vi "Populate Database Table.vi"() -> ()   [LabVIEW 2019]
uses:
  Controls/Table Data Types/Inventory Data Type.ctl
  Controls/Table Data Types/User Data Type.ctl
  Controls/Table Data Types/Inventory Archive Data Type.ctl
  Controls/Table Data Types/User Archive Data Type.ctl
  Controls/Table Data Types/Checked In Archive Data Type.ctl
  <vilib>/addons/database/Connection.llb/DB Tools Open Connec (String).vi
  <vilib>/Utility/file.llb/Read Delimited Spreadsheet (string).vi
  <vilib>/addons/database/NI_Database_API.lvlib
panel:
  in  "Checked In TXT File":path
  in  "User Archive TXT File":path
  in  "Inventory Archive TXT File":path
  in  "User TXT File":path
  in  "Inventory TXT File":path
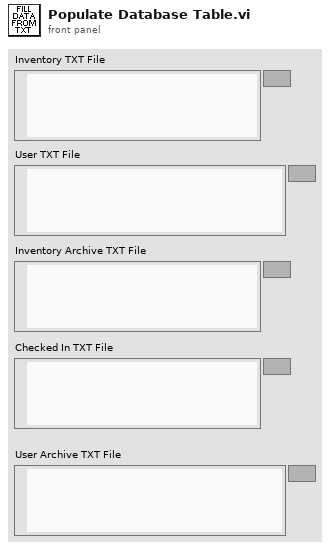
[diagram p1: front panel]
types:
  T1 = typedef "NI_Database_API.lvlib/Conn ObjectReference.ctl" = refnum<k1>
  T2 = typedef "Inventory Data Type.ctl" = cluster{"Identifier":string, "BYU ICN #":string, "Item Description":string, "Comments":string, "Checked Out Date":string, "Due Date":string, "Check Out Location":string, "Reminder Count":i32, "Most Recent Reminder Date":string, "BYU ID #":string, "Building/Room":string, "Location in Room":string, "Manual":string, "Manufacturer":string, "Model #":string, "Serial #":string, "Date Acquired":string}
  T3 = typedef "User Data Type.ctl" = cluster{"BYU ID #":string, "First Name":string, "Last Name":string, "Phone Number":string, "Email":string, "Department":string, "Graduation Status":string, "Anticipated Graduation Year":string, "Credit Score":dbl, "Date Added":string, "Graduation Clearance Date":string, "Picture File Name":string}
  T4 = typedef "Inventory Archive Data Type.ctl" = cluster{"Date Disposed":string, "Disposal Method":string, "Auction #":string, "Date Inventory Office Emailed":string, "Disposal Notes":string, "Identifier":string, "BYU ICN #":string, "Item Description":string, "Comments":string, "Building/Room":string, "Location in Room":string, "Manual":string, "Manufacturer":string, "Model #":string, "Serial #":string, "Date Acquired":string}
  T5 = typedef "User Archive Data Type.ctl" = cluster{"BYU ID #":string, "First Name":string, "Last Name":string, "Phone Number":string, "Email":string, "Department":string, "Graduation Status":string, "Anticipated Graduation Year":string, "Credit Score":dbl, "Date Added":string, "Graduation Clearance Date":string, "Picture File Name":string, "Date Archived":string}
  T6 = typedef "Checked In Archive Data Type.ctl" = cluster{"Identifier":string, "BYU ICN #":string, "Item Description":string, "Comments":string, "Checked Out Date":string, "Due Date":string, "Check Out Location":string, "Reminder Count":i32, "Most Recent Reminder Date":string, "BYU ID #":string, "Building/Room":string, "Location in Room":string, "Manual":string, "Manufacturer":string, "Model #":string, "Serial #":string, "Date Acquired":string, "Date Returned":string}
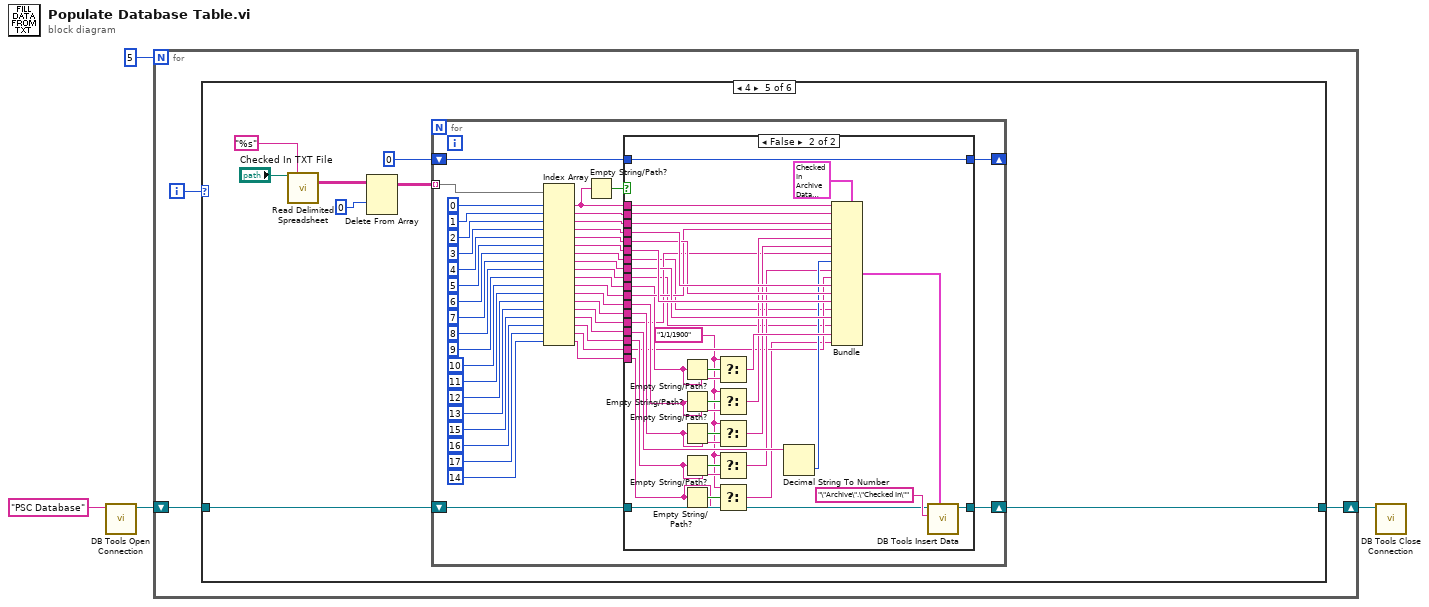
[diagram p0: block diagram]
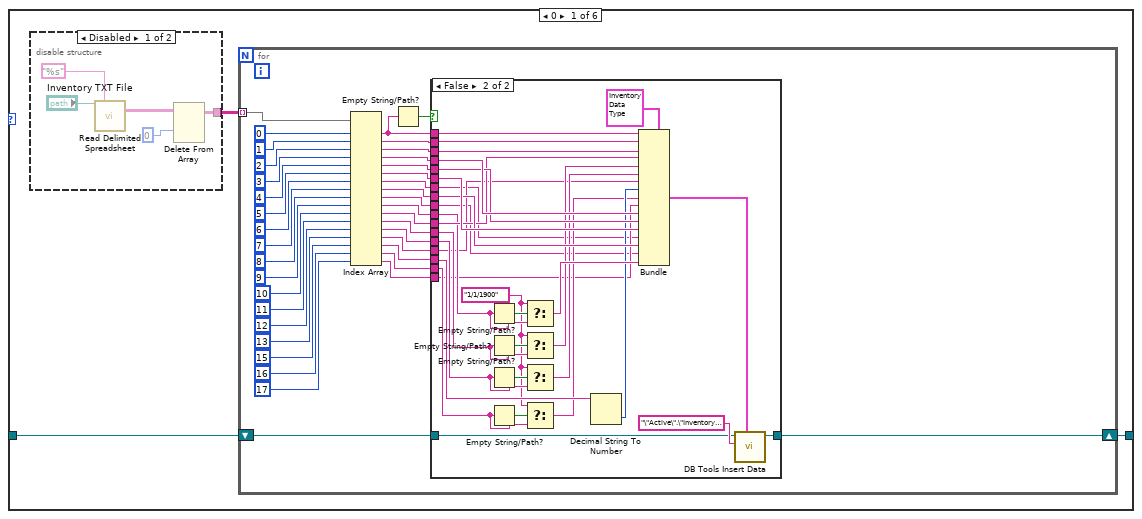
[diagram p2: hidden frame]
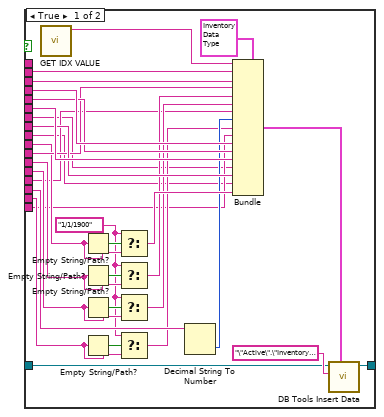
[diagram p4: hidden frame]
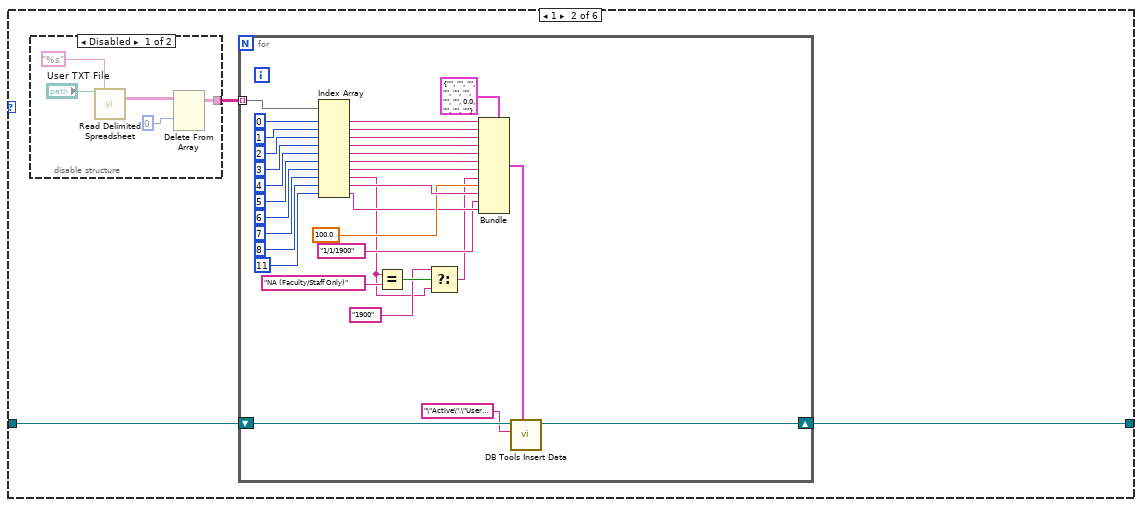
[diagram p5: hidden frame]
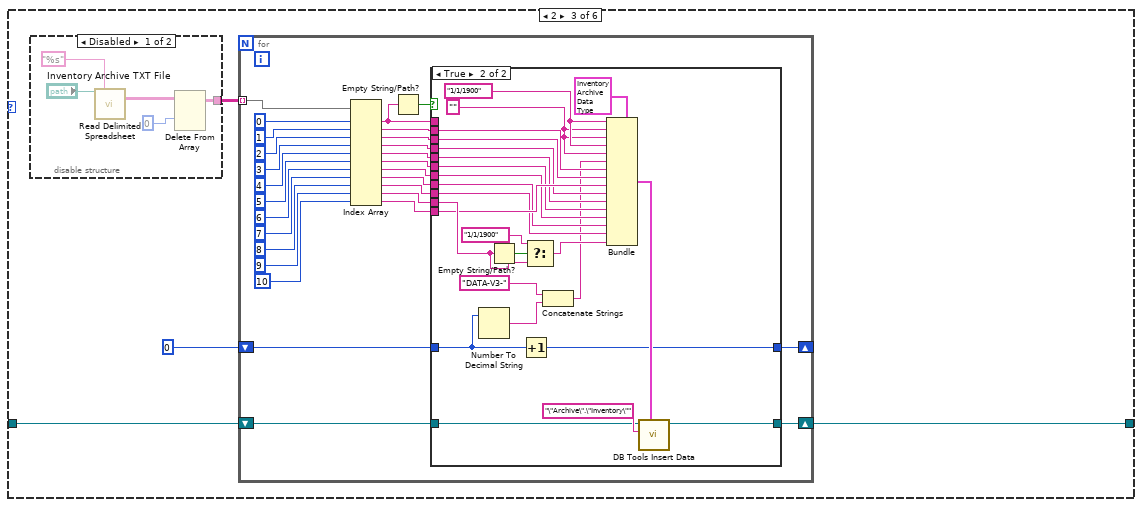
[diagram p7: hidden frame]
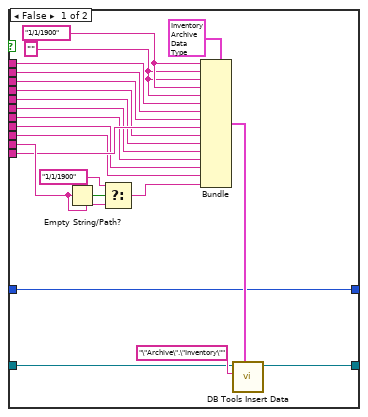
[diagram p9: hidden frame]
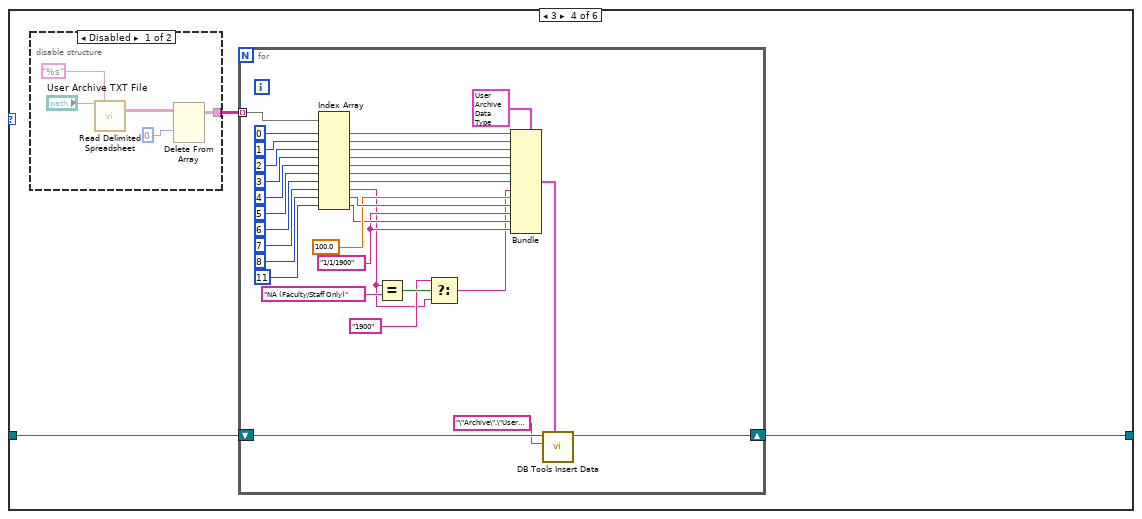
[diagram p10: hidden frame]
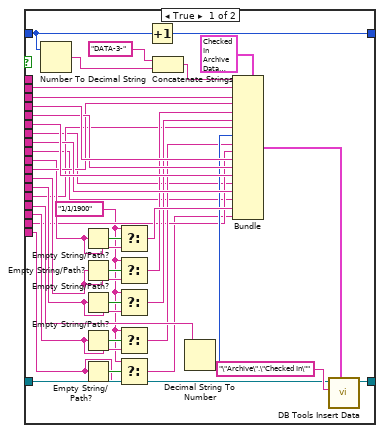
[diagram p12: hidden frame]
diagram:
  n1 = call-poly <vilib>:"DB Tools Open Connection.vi"("connection information"="PSC Database") -> ("connection reference"=w3:T1)  [unwired: 7 in, 1 out]
  n2 = for {
    N: 5 -> [_]
    shift-right: [w5] -> w1
    shift-left: w3 -> [w7]
    i -> [w6]
    n3 = case shown="4" w6 {
      tunnel: w7 -> [w10 w120 w161 w244 w287 w407]
      tunnel: [w9 w119 w160 w243 w286 w407] -> w5
      frame 0 {
        n4 = disable-structure shown="Disabled" {
          disable-tunnel: [w11 _] -> w8
          frame Disabled {
            n5 = call-poly <vilib>:"Read Delimited Spreadsheet.vi"("file path (dialog if empty)"="Inventory TXT File", "format (%s)"="%s") -> ("all rows"=w12:string[][])  [unwired: 8 in, 5 out]
            n6 = Delete From Array(array=w12, index (row)=0) -> (array with subset deleted=w11:string[][])  [unwired: 2 in, 1 out]
          }
          frame Enabled {
          }
        }
        n7 = for {
          tunnel: w8 -> [w53] mode=indexing
          shift-right: [w16] -> w9
          shift-left: w10 -> [w34]
          n8 = Index Array(array=w53, index #1=0 ("index"), index #2=1 ("index"), index #3=2 ("index"), index #4=3 ("index"), index #5=4 ("index"), index #6=5 ("index"), index #7=6 ("index"), index #8=7 ("index"), index #9=8 ("index"), index #10=9 ("index"), index #11=10 ("index"), index #12=11 ("index"), index #13=12 ("index"), index #14=13 ("index"), index #15=15 ("index"), index #16=16 ("index"), index #17=17 ("index")) -> (element #1=w27:string, element #2=w33:string, element #3=w32:string, element #4=w31:string, element #5=w30:string, element #6=w29:string, element #7=w28:string, element #8=w26:string, element #9=w25:string, element #10=w24:string, element #11=w23:string, element #12=w22:string, element #13=w21:string, element #14=w20:string, element #15=w19:string, element #16=w18:string, element #17=w17:string)
          n9 = Empty String/Path?(string/path=w27) -> (empty?=w35:bool)
          n10 = case shown="False" w35 {
            tunnel: w34 -> [w55 w88]
            tunnel: w33 -> [w83 w115]
            tunnel: w32 -> [w82 w114]
            tunnel: w31 -> [w81 w113]
            tunnel: w30 -> [w80 w112]
            tunnel: w29 -> [w79 w111]
            tunnel: w28 -> [w57 w90]
            tunnel: w27 -> [_ w87]
            tunnel: w26 -> [w78 w110]
            tunnel: w25 -> [w58 w91]
            tunnel: w24 -> [w74 w107]
            tunnel: w23 -> [w76 w109]
            tunnel: w22 -> [w72 w105]
            tunnel: w21 -> [w70 w103]
            tunnel: w20 -> [w66 w99]
            tunnel: w19 -> [w65 w98]
            tunnel: w18 -> [w62 w95]
            tunnel: w17 -> [w59 w92]
            tunnel: [w54 w86] -> w16
            frame True {
              w61 = "1/1/1900"
              n11 = call "GET IDX VALUE.vi"() -> ("Identifier Out"=w77:string)  [unwired: 11 in]
              n12 = Empty String/Path?(string/path=w74) -> (empty?=w75:bool)
              n13 = Empty String/Path?(string/path=w72) -> (empty?=w73:bool)
              n14 = Empty String/Path?(string/path=w70) -> (empty?=w71:bool)
              n15 = Empty String/Path?(string/path=w62) -> (empty?=w63:bool)
              n16 = Select(t=w61, s=w75, f=w74) -> (s? t:f=w69:string)
              n17 = Select(t=w61, s=w73, f=w72) -> (s? t:f=w68:string)
              n18 = Select(t=w61, s=w71, f=w70) -> (s? t:f=w67:string)
              n19 = Select(t=w61, s=w63, f=w62) -> (s? t:f=w60:string)
              n20 = Decimal String To Number(string=w65) -> (number=w64:i32)  [unwired: 2 in, 1 out]
              n21 = Bundle(cluster=T2 {"Identifier"="", "BYU ICN #"="", "Item Description"="", "Comments"="", "Checked Out Date"="", "Due Date"="", "Check Out Location"="", "Reminder Count"=0, "Most Recent Reminder Date"="", "BYU ID #"="", "Building/Room"="", "Location in Room"="", "Manual"="", "Manufacturer"="", "Model #"="", "Serial #"="", "Date Acquired"=""} ("INVENTORY DATA TYPE"), "Identifier"=w77, "BYU ICN #"=w83, "Item Description"=w82, "Comments"=w76, "Checked Out Date"=w68, "Due Date"=w67, "Check Out Location"=w66, "Reminder Count"=w64, "Most Recent Reminder Date"=w60, "BYU ID #"=w59, "Building/Room"=w81, "Location in Room"=w80, "Manual"=w79, "Manufacturer"=w57, "Model #"=w78, "Serial #"=w58, "Date Acquired"=w69) -> (w56:T2)
              n22 = call <vilib>:"DB Tools Insert Data.vi"("data"=w56, "table"="\"Active\".\"Inventory\"", "connection reference"=w55) -> ("connection reference out"=w54:T1)  [unwired: 7 in, 1 out]
            }
            frame False {
              w94 = "1/1/1900"
              n23 = Empty String/Path?(string/path=w107) -> (empty?=w108:bool)
              n24 = Empty String/Path?(string/path=w105) -> (empty?=w106:bool)
              n25 = Empty String/Path?(string/path=w103) -> (empty?=w104:bool)
              n26 = Empty String/Path?(string/path=w95) -> (empty?=w96:bool)
              n27 = Select(t=w94, s=w108, f=w107) -> (s? t:f=w102:string)
              n28 = Select(t=w94, s=w106, f=w105) -> (s? t:f=w101:string)
              n29 = Select(t=w94, s=w104, f=w103) -> (s? t:f=w100:string)
              n30 = Select(t=w94, s=w96, f=w95) -> (s? t:f=w93:string)
              n31 = Decimal String To Number(string=w98) -> (number=w97:i32)  [unwired: 2 in, 1 out]
              n32 = Bundle(cluster=T2 {"Identifier"="", "BYU ICN #"="", "Item Description"="", "Comments"="", "Checked Out Date"="", "Due Date"="", "Check Out Location"="", "Reminder Count"=0, "Most Recent Reminder Date"="", "BYU ID #"="", "Building/Room"="", "Location in Room"="", "Manual"="", "Manufacturer"="", "Model #"="", "Serial #"="", "Date Acquired"=""} ("INVENTORY DATA TYPE"), "Identifier"=w87, "BYU ICN #"=w115, "Item Description"=w114, "Comments"=w109, "Checked Out Date"=w101, "Due Date"=w100, "Check Out Location"=w99, "Reminder Count"=w97, "Most Recent Reminder Date"=w93, "BYU ID #"=w92, "Building/Room"=w113, "Location in Room"=w112, "Manual"=w111, "Manufacturer"=w90, "Model #"=w110, "Serial #"=w91, "Date Acquired"=w102) -> (w89:T2)
              n33 = call <vilib>:"DB Tools Insert Data.vi"("data"=w89, "table"="\"Active\".\"Inventory\"", "connection reference"=w88) -> ("connection reference out"=w86:T1)  [unwired: 7 in, 1 out]
            }
          }
        }
      }
      frame 1 {
        n34 = disable-structure shown="Disabled" {
          disable-tunnel: [w121 _] -> w118
          frame Disabled {
            n35 = call-poly <vilib>:"Read Delimited Spreadsheet.vi"("file path (dialog if empty)"="User TXT File", "format (%s)"="%s") -> ("all rows"=w122:string[][])  [unwired: 8 in, 5 out]
            n36 = Delete From Array(array=w122, index (row)=0) -> (array with subset deleted=w121:string[][])  [unwired: 2 in, 1 out]
          }
          frame Enabled {
          }
        }
        n37 = for {
          tunnel: w118 -> [w157] mode=indexing
          shift-right: [w145] -> w119
          shift-left: w120 -> [w146]
          n38 = Index Array(array=w157, index #1=0 ("index"), index #2=1 ("index"), index #3=2 ("index"), index #4=3 ("index"), index #5=4 ("index"), index #6=5 ("index"), index #7=6 ("index"), index #8=7 ("index"), index #9=8 ("index"), index #10=11 ("index")) -> (element #1=w141:string, element #2=w140:string, element #3=w139:string, element #4=w138:string, element #5=w137:string, element #6=w136:string, element #7=w135:string, element #8=w127:string, element #9=w134:string, element #10=w132:string)
          n39 = Equal?(x=w127, y="NA (Faculty/Staff Only)" ("Graduation Clearance Date")) -> (x = y?=w129:bool)
          n40 = Select(t="1900" ("Graduation Clearance Date"), s=w129, f=w127) -> (s? t:f=w126:string)
          n41 = Bundle(cluster=T3 {"BYU ID #"="", "First Name"="", "Last Name"="", "Phone Number"="", "Email"="", "Department"="", "Graduation Status"="", "Anticipated Graduation Year"="", "Credit Score"=0.0, "Date Added"="", "Graduation Clearance Date"="", "Picture File Name"=""} ("USER DATA TYPE"), "BYU ID #"=w141, "First Name"=w140, "Last Name"=w139, "Phone Number"=w138, "Email"=w137, "Department"=w136, "Graduation Status"=w135, "Anticipated Graduation Year"=w126, "Credit Score"=100.0, "Date Added"=w134, "Graduation Clearance Date"="1/1/1900", "Picture File Name"=w132) -> (w143:T3)
          n42 = call <vilib>:"DB Tools Insert Data.vi"("data"=w143, "table"="\"Active\".\"Users\"", "connection reference"=w146) -> ("connection reference out"=w145:T1)  [unwired: 7 in, 1 out]
        }
      }
      frame 2 {
        n43 = disable-structure shown="Disabled" {
          disable-tunnel: [w163 _] -> w158
          frame Disabled {
            n44 = call-poly <vilib>:"Read Delimited Spreadsheet.vi"("file path (dialog if empty)"="Inventory Archive TXT File", "format (%s)"="%s") -> ("all rows"=w164:string[][])  [unwired: 8 in, 5 out]
            n45 = Delete From Array(array=w164, index (row)=0) -> (array with subset deleted=w163:string[][])  [unwired: 2 in, 1 out]
          }
          frame Enabled {
          }
        }
        n46 = for {
          tunnel: w158 -> [w194] mode=indexing
          shift-right: [w169] -> w160
          shift-left: w161 -> [w181]
          shift-right: [w167] -> _
          shift-left: 0 -> [w168]
          n47 = Index Array(array=w194, index #1=0 ("index"), index #2=1 ("index"), index #3=2 ("index"), index #4=3 ("index"), index #5=4 ("index"), index #6=5 ("index"), index #7=6 ("index"), index #8=7 ("index"), index #9=8 ("index"), index #10=9 ("index"), index #11=10 ("index")) -> (element #1=w174:string, element #2=w180:string, element #3=w179:string, element #4=w178:string, element #5=w177:string, element #6=w176:string, element #7=w175:string, element #8=w173:string, element #9=w172:string, element #10=w171:string, element #11=w170:string)
          n48 = Empty String/Path?(string/path=w174) -> (empty?=w182:bool)
          n49 = case shown="True" w182 {
            tunnel: w181 -> [w211 w236]
            tunnel: w180 -> [w205 w231]
            tunnel: w179 -> [w204 w230]
            tunnel: w178 -> [w202 w228]
            tunnel: w177 -> [w201 w227]
            tunnel: w176 -> [w200 w226]
            tunnel: w175 -> [w199 w225]
            tunnel: w174 -> [w208 _]
            tunnel: w173 -> [w198 w224]
            tunnel: w172 -> [w197 w223]
            tunnel: w171 -> [w214 w239]
            tunnel: w170 -> [w203 w229]
            tunnel: [w210 w235] -> w169
            tunnel: w168 -> [w195 w218]
            tunnel: [w195 w217] -> w167
            frame False {
              w206 = "" ("Disposal Method")
              w207 = "1/1/1900"
              n50 = Empty String/Path?(string/path=w214) -> (empty?=w215:bool)
              n51 = Select(t="1/1/1900", s=w215, f=w214) -> (s? t:f=w196:string)
              n52 = Bundle(cluster=T4 {"Date Disposed"="", "Disposal Method"="", "Auction #"="", "Date Inventory Office Emailed"="", "Disposal Notes"="", "Identifier"="", "BYU ICN #"="", "Item Description"="", "Comments"="", "Building/Room"="", "Location in Room"="", "Manual"="", "Manufacturer"="", "Model #"="", "Serial #"="", "Date Acquired"=""} ("INVENTORY ARCHIVE DATA TYPE"), "Date Disposed"=w207, "Disposal Method"=w206, "Auction #"=w206, "Date Inventory Office Emailed"=w207, "Disposal Notes"=w206, "Identifier"=w208, "BYU ICN #"=w205, "Item Description"=w204, "Comments"=w203, "Building/Room"=w202, "Location in Room"=w201, "Manual"=w200, "Manufacturer"=w199, "Model #"=w198, "Serial #"=w197, "Date Acquired"=w196) -> (w212:T4)
              n53 = call <vilib>:"DB Tools Insert Data.vi"("data"=w212, "table"="\"Archive\".\"Inventory\"", "connection reference"=w211) -> ("connection reference out"=w210:T1)  [unwired: 7 in, 1 out]
            }
            frame True {
              w232 = "" ("Disposal Method")
              w233 = "1/1/1900"
              n54 = Number To Decimal String(number=w218) -> (decimal integer string=w220:string)  [unwired: 1 in]
              n55 = Empty String/Path?(string/path=w239) -> (empty?=w240:bool)
              n56 = Increment(x=w218) -> (x+1=w217:i32)
              n57 = Select(t="1/1/1900", s=w240, f=w239) -> (s? t:f=w222:string)
              n58 = Concatenate Strings("DATA-V3-" ("Identifier"), w220) -> (w219:string)
              n59 = Bundle(cluster=T4 {"Date Disposed"="", "Disposal Method"="", "Auction #"="", "Date Inventory Office Emailed"="", "Disposal Notes"="", "Identifier"="", "BYU ICN #"="", "Item Description"="", "Comments"="", "Building/Room"="", "Location in Room"="", "Manual"="", "Manufacturer"="", "Model #"="", "Serial #"="", "Date Acquired"=""} ("INVENTORY ARCHIVE DATA TYPE"), "Date Disposed"=w233, "Disposal Method"=w232, "Auction #"=w232, "Date Inventory Office Emailed"=w233, "Disposal Notes"=w232, "Identifier"=w219, "BYU ICN #"=w231, "Item Description"=w230, "Comments"=w229, "Building/Room"=w228, "Location in Room"=w227, "Manual"=w226, "Manufacturer"=w225, "Model #"=w224, "Serial #"=w223, "Date Acquired"=w222) -> (w237:T4)
              n60 = call <vilib>:"DB Tools Insert Data.vi"("data"=w237, "table"="\"Archive\".\"Inventory\"", "connection reference"=w236) -> ("connection reference out"=w235:T1)  [unwired: 7 in, 1 out]
            }
          }
        }
      }
      frame 3 {
        n61 = disable-structure shown="Disabled" {
          disable-tunnel: [w245 _] -> w242
          frame Disabled {
            n62 = call-poly <vilib>:"Read Delimited Spreadsheet.vi"("file path (dialog if empty)"="User Archive TXT File", "format (%s)"="%s") -> ("all rows"=w246:string[][])  [unwired: 8 in, 5 out]
            n63 = Delete From Array(array=w246, index (row)=0) -> (array with subset deleted=w245:string[][])  [unwired: 2 in, 1 out]
          }
          frame Enabled {
          }
        }
        n64 = for {
          tunnel: w242 -> [w281] mode=indexing
          shift-right: [w269] -> w243
          shift-left: w244 -> [w270]
          w255 = "1/1/1900" ("Graduation Clearance Date")
          n65 = Index Array(array=w281, index #1=0 ("index"), index #2=1 ("index"), index #3=2 ("index"), index #4=3 ("index"), index #5=4 ("index"), index #6=5 ("index"), index #7=6 ("index"), index #8=7 ("index"), index #9=8 ("index"), index #10=11 ("index")) -> (element #1=w266:string, element #2=w265:string, element #3=w264:string, element #4=w263:string, element #5=w262:string, element #6=w261:string, element #7=w260:string, element #8=w250:string, element #9=w259:string, element #10=w257:string)
          n66 = Equal?(x=w250, y="NA (Faculty/Staff Only)" ("Graduation Clearance Date")) -> (x = y?=w254:bool)
          n67 = Select(t="1900" ("Graduation Clearance Date"), s=w254, f=w250) -> (s? t:f=w251:string)
          n68 = Bundle(cluster=T5 {"BYU ID #"="", "First Name"="", "Last Name"="", "Phone Number"="", "Email"="", "Department"="", "Graduation Status"="", "Anticipated Graduation Year"="", "Credit Score"=0.0, "Date Added"="", "Graduation Clearance Date"="", "Picture File Name"="", "Date Archived"=""} ("USER ARCHIVE DATA TYPE"), "BYU ID #"=w266, "First Name"=w265, "Last Name"=w264, "Phone Number"=w263, "Email"=w262, "Department"=w261, "Graduation Status"=w260, "Anticipated Graduation Year"=w251, "Credit Score"=100.0, "Date Added"=w259, "Graduation Clearance Date"=w255, "Picture File Name"=w257, "Date Archived"=w255) -> (w267:T5)
          n69 = call <vilib>:"DB Tools Insert Data.vi"("data"=w267, "table"="\"Archive\".\"Users\"", "connection reference"=w270) -> ("connection reference out"=w269:T1)  [unwired: 7 in, 1 out]
        }
      }
      frame 4 {
        n70 = call-poly <vilib>:"Read Delimited Spreadsheet.vi"("file path (dialog if empty)"="Checked In TXT File", "format (%s)"="%s") -> ("all rows"=w284:string[][])  [unwired: 8 in, 5 out]
        n71 = Delete From Array(array=w284, index (row)=0) -> (array with subset deleted=w283:string[][])  [unwired: 2 in, 1 out]
        n72 = for {
          tunnel: w283 -> [w331] mode=indexing
          shift-right: [w294] -> w286
          shift-left: w287 -> [w312]
          shift-right: [w290] -> _
          shift-left: 0 -> [w293]
          n73 = Index Array(array=w331, index #1=0 ("index"), index #2=1 ("index"), index #3=2 ("index"), index #4=3 ("index"), index #5=4 ("index"), index #6=5 ("index"), index #7=6 ("index"), index #8=7 ("index"), index #9=8 ("index"), index #10=9 ("index"), index #11=10 ("index"), index #12=11 ("index"), index #13=12 ("index"), index #14=13 ("index"), index #15=15 ("index"), index #16=16 ("index"), index #17=17 ("index"), index #18=14 ("index")) -> (element #1=w305:string, element #2=w311:string, element #3=w310:string, element #4=w309:string, element #5=w308:string, element #6=w307:string, element #7=w306:string, element #8=w304:string, element #9=w303:string, element #10=w302:string, element #11=w301:string, element #12=w300:string, element #13=w299:string, element #14=w298:string, element #15=w297:string, element #16=w296:string, element #17=w295:string, element #18=w291:string)
          n74 = Empty String/Path?(string/path=w305) -> (empty?=w313:bool)
          n75 = case shown="False" w313 {
            tunnel: w312 -> [w343 w379]
            tunnel: w311 -> [w369 w405]
            tunnel: w310 -> [w368 w404]
            tunnel: w309 -> [w367 w403]
            tunnel: w308 -> [w366 w402]
            tunnel: w307 -> [w365 w401]
            tunnel: w306 -> [w345 w381]
            tunnel: w305 -> [_ w378]
            tunnel: w304 -> [w364 w400]
            tunnel: w303 -> [w346 w382]
            tunnel: w302 -> [w361 w397]
            tunnel: w301 -> [w363 w399]
            tunnel: w300 -> [w359 w395]
            tunnel: w299 -> [w357 w393]
            tunnel: w298 -> [w353 w389]
            tunnel: w297 -> [w352 w388]
            tunnel: w296 -> [w349 w385]
            tunnel: w295 -> [w347 w383]
            tunnel: [w342 w377] -> w294
            tunnel: w293 -> [w333 w371]
            tunnel: w291 -> [w336 w372]
            tunnel: [w332 w371] -> w290
            frame True {
              w334 = "1/1/1900"
              n76 = Number To Decimal String(number=w333) -> (decimal integer string=w340:string)  [unwired: 1 in]
              n77 = Empty String/Path?(string/path=w361) -> (empty?=w362:bool)
              n78 = Empty String/Path?(string/path=w359) -> (empty?=w360:bool)
              n79 = Empty String/Path?(string/path=w357) -> (empty?=w358:bool)
              n80 = Empty String/Path?(string/path=w349) -> (empty?=w350:bool)
              n81 = Empty String/Path?(string/path=w336) -> (empty?=w337:bool)
              n82 = Select(t=w334, s=w362, f=w361) -> (s? t:f=w356:string)
              n83 = Select(t=w334, s=w360, f=w359) -> (s? t:f=w355:string)
              n84 = Select(t=w334, s=w358, f=w357) -> (s? t:f=w354:string)
              n85 = Select(t=w334, s=w350, f=w349) -> (s? t:f=w348:string)
              n86 = Select(t=w334, s=w337, f=w336) -> (s? t:f=w335:string)
              n87 = Increment(x=w333) -> (x+1=w332:i32)
              n88 = Concatenate Strings("DATA-3-", w340) -> (w339:string)
              n89 = Decimal String To Number(string=w352) -> (number=w351:i32)  [unwired: 2 in, 1 out]
              n90 = Bundle(cluster=T6 {"Identifier"="", "BYU ICN #"="", "Item Description"="", "Comments"="", "Checked Out Date"="", "Due Date"="", "Check Out Location"="", "Reminder Count"=0, "Most Recent Reminder Date"="", "BYU ID #"="", "Building/Room"="", "Location in Room"="", "Manual"="", "Manufacturer"="", "Model #"="", "Serial #"="", "Date Acquired"="", "Date Returned"=""} ("CHECKED IN ARCHIVE DATA TYPE"), "Identifier"=w339, "BYU ICN #"=w369, "Item Description"=w368, "Comments"=w363, "Checked Out Date"=w355, "Due Date"=w354, "Check Out Location"=w353, "Reminder Count"=w351, "Most Recent Reminder Date"=w348, "BYU ID #"=w347, "Building/Room"=w367, "Location in Room"=w366, "Manual"=w365, "Manufacturer"=w345, "Model #"=w364, "Serial #"=w346, "Date Acquired"=w356, "Date Returned"=w335) -> (w344:T6)
              n91 = call <vilib>:"DB Tools Insert Data.vi"("data"=w344, "table"="\"Archive\".\"Checked In\"", "connection reference"=w343) -> ("connection reference out"=w342:T1)  [unwired: 7 in, 1 out]
            }
            frame False {
              w373 = "1/1/1900"
              n92 = Empty String/Path?(string/path=w397) -> (empty?=w398:bool)
              n93 = Empty String/Path?(string/path=w395) -> (empty?=w396:bool)
              n94 = Empty String/Path?(string/path=w393) -> (empty?=w394:bool)
              n95 = Empty String/Path?(string/path=w385) -> (empty?=w386:bool)
              n96 = Empty String/Path?(string/path=w372) -> (empty?=w375:bool)
              n97 = Select(t=w373, s=w398, f=w397) -> (s? t:f=w392:string)
              n98 = Select(t=w373, s=w396, f=w395) -> (s? t:f=w391:string)
              n99 = Select(t=w373, s=w394, f=w393) -> (s? t:f=w390:string)
              n100 = Select(t=w373, s=w386, f=w385) -> (s? t:f=w384:string)
              n101 = Select(t=w373, s=w375, f=w372) -> (s? t:f=w374:string)
              n102 = Decimal String To Number(string=w388) -> (number=w387:i32)  [unwired: 2 in, 1 out]
              n103 = Bundle(cluster=T6 {"Identifier"="", "BYU ICN #"="", "Item Description"="", "Comments"="", "Checked Out Date"="", "Due Date"="", "Check Out Location"="", "Reminder Count"=0, "Most Recent Reminder Date"="", "BYU ID #"="", "Building/Room"="", "Location in Room"="", "Manual"="", "Manufacturer"="", "Model #"="", "Serial #"="", "Date Acquired"="", "Date Returned"=""} ("CHECKED IN ARCHIVE DATA TYPE"), "Identifier"=w378, "BYU ICN #"=w405, "Item Description"=w404, "Comments"=w399, "Checked Out Date"=w391, "Due Date"=w390, "Check Out Location"=w389, "Reminder Count"=w387, "Most Recent Reminder Date"=w384, "BYU ID #"=w383, "Building/Room"=w403, "Location in Room"=w402, "Manual"=w401, "Manufacturer"=w381, "Model #"=w400, "Serial #"=w382, "Date Acquired"=w392, "Date Returned"=w374) -> (w380:T6)
              n104 = call <vilib>:"DB Tools Insert Data.vi"("data"=w380, "table"="\"Archive\".\"Checked In\"", "connection reference"=w379) -> ("connection reference out"=w377:T1)  [unwired: 7 in, 1 out]
            }
          }
        }
      }
      frame Default {
      }
    }
  }
  n105 = call <vilib>:"DB Tools Close Connection.vi"("connection reference"=w1) -> ()  [unwired: 6 in, 1 out]
